vi "Example Client.vi"() -> ()   [LabVIEW 2018, in "TCPServer.lvlib"]
uses:
  TCPServer.lvlib
  TypeDefs/CCSDS.ctl
  TypeDefs/Sec Hdr CMD.ctl
  TypeDefs/Sec Hdr TLM.ctl
  d66480fc-37c9-4712-92ef-9cdd99e438f4.vi
panel:
  in  "CMD in":cluster{"U8":u8, "DBL":dbl}={"U8"=2, "DBL"=3.14}
  out "TLM out":cluster{"VOLTAGE":dbl, "NAME[20]":string}
  out "TLM Length":i32
  out "TLM Packet":string
  in  "CMD ID":u8=1
  in  "error in (no error)":errorcluster
  out "error out":errorcluster
  out "CMD Packet":string
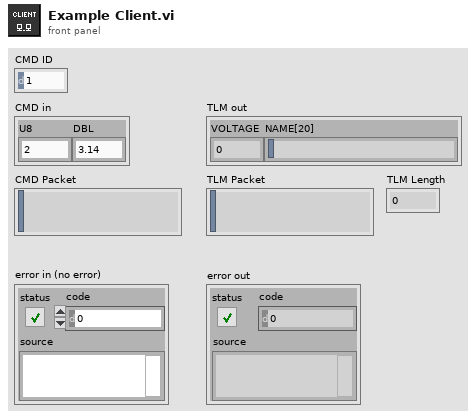
[diagram p1: front panel]
types:
  T1 = typedef "TCPServer.lvlib/Sec Hdr TLM.ctl" = cluster{"DAYS_SINCE_2000":u16, "SECONDS_SINCE_START":u32, "MS_SINCE_START":u16}
  T2 = typedef "TCPServer.lvlib/Sec Hdr CMD.ctl" = cluster{"CMD_ID":u8, "CMD_CHECKSUM":u8}
  T3 = typedef "TCPServer.lvlib/CCSDS.ctl" = cluster{"Version":u8, "Type":enum8{"TLM", "CMD"}, "SecHdrFlag":bool, "AppID":u16, "SeqFlags":u8, "SeqCount":u16, "PktLength":u16}
  T4 = cluster{"HDR_TYPE":u16, "HDR_SEQ":u16, "HDR_LENGTH":u16}
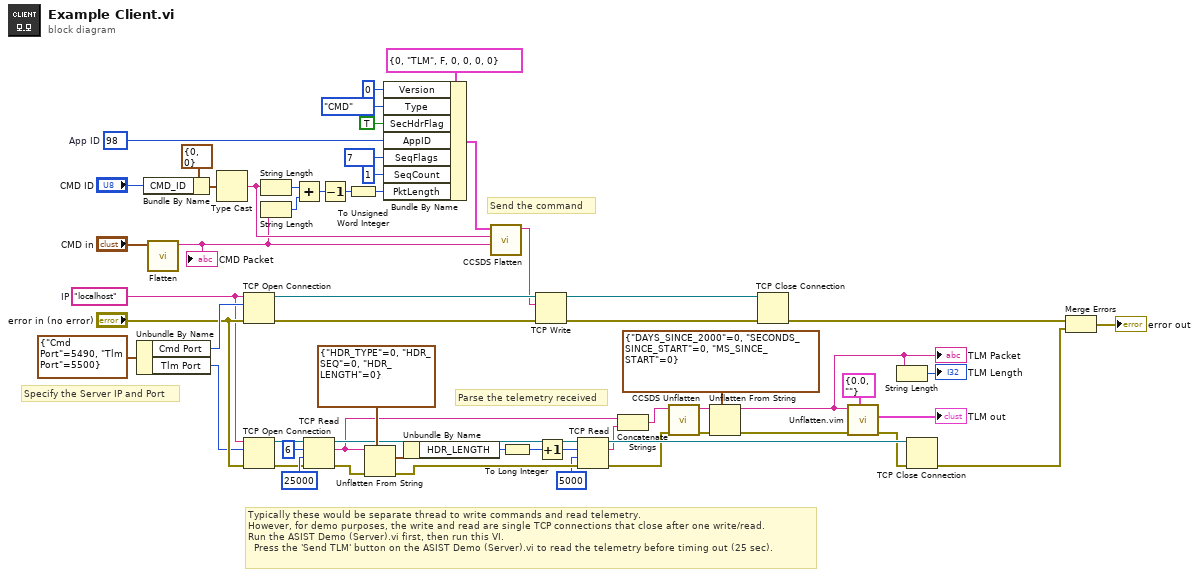
[diagram p0: block diagram]
diagram:
  w20 = u16 98  # App ID
  w16 = "localhost"  # IP
  # "Send the command"
  # "Parse the telemetry received"
  # "Typically these would be separate thread to write commands and read telemetry.\nHowever, for demo purposes, the write and read are single TCP connections that close after one write/read.\nRun the ASIST Demo (Server).vi first, then run this VI.\n  Press the 'Send TLM' button on the ASIST Demo (Server).vi to read the telemetry before timing out (25 sec)."
  # "Specify the Server IP and Port"
  n1 = Unbundle By Name(cluster{"Cmd Port":u16, "Tlm Port":u16} {"Cmd Port"=5490, "Tlm Port"=5500} ("Ports")) -> ("Cmd Port"=w18:u16, "Tlm Port"=w15:u16)
  n2 = Bundle By Name(cluster=T2 {"CMD_ID"=0, "CMD_CHECKSUM"=0} ("CCSDS Secondary Header in"), "CMD_ID"="CMD ID") -> (w32:T2)
  n3 = call "Flatten.vi"("Cluster"="CMD in") -> ("String"=w6:string)  [unwired: 9 in, 1 out]
  "CMD Packet" <- w6
  n4 = Type Cast(x=w32) -> (*(type *) &x=w31:string)  [unwired: 1 in]
  n5 = TCP Open Connection(address=w16, remote port or service name=w18, error in (no error)="error in (no error)") -> (connection ID=w59:refnum<k5>, error out=w58:errorcluster)  [unwired: 2 in]
  n6 = TCP Open Connection(address=w16, remote port or service name=w15, error in (no error)="error in (no error)") -> (connection ID=w13:refnum<k5>, error out=w14:errorcluster)  [unwired: 2 in]
  n7 = String Length(string=w31) -> (length=w37:i32)
  n8 = String Length(string=w6) -> (length=w36:i32)
  n9 = Add(x=w37, y=w36) -> (x+y=w35:i32)
  n10 = TCP Read(connection ID=w13, bytes to read=6, error in (no error)=w14, 9:25000 ("timeout ms (25000)")) -> (connection ID out=w45:refnum<k5>, data out=w43:string, error out=w53:errorcluster)  [unwired: 1 in]
  n11 = Decrement(x=w35) -> (x-1=w33:i32)
  n12 = To Unsigned Word Integer(number=w33) -> (unsigned 16bit integer=w34:u16)
  n13 = Unflatten From String(type=T4 {"HDR_TYPE"=0, "HDR_SEQ"=0, "HDR_LENGTH"=0} ("ASIST"), binary string=w43, error in (no error)=w53) -> (value=w50:T4, error out=w51:errorcluster)  [unwired: 2 in, 1 out]
  n14 = Bundle By Name(cluster=T3 {"Version"=0, "Type"=enum."TLM", "SecHdrFlag"=FALSE, "AppID"=0, "SeqFlags"=0, "SeqCount"=0, "PktLength"=0} ("CCSDS Primary Header in"), "Version"=u8 0, "Type"=enum8{"TLM", "CMD"}."CMD", "SecHdrFlag"=TRUE, "AppID"=w20, "SeqFlags"=u8 7, "SeqCount"=u16 1, "PktLength"=w34) -> (w38:T3)
  n15 = Unbundle By Name(w50) -> ("HDR_LENGTH"=w49:u16)
  n16 = call "CCSDS Flatten.vi"("Packet Data in"=w6, "Secondary Header in"=w31, "CCSDS Primary Header in"=w38) -> ("CCSDS Packet out"=w39:string)  [unwired: 7 in, 1 out]
  n17 = To Long Integer(number=w49) -> (32bit integer=w48:i32)
  n18 = TCP Write(connection ID=w59, data in=w39, error in (no error)=w58) -> (connection ID out=w11:refnum<k5>, error out=w12:errorcluster)  [unwired: 1 in, 1 out]
  n19 = Increment(x=w48) -> (x+1=w40:i32)
  n20 = TCP Read(connection ID=w45, bytes to read=w40, error in (no error)=w51, 9:5000 ("timeout ms (25000)")) -> (connection ID out=w55:refnum<k5>, data out=w44:string, error out=w42:errorcluster)  [unwired: 1 in]
  n21 = Concatenate Strings(w43, w44) -> (w41:string)
  n22 = call "CCSDS Unflatten.vi"("error in (no error)"=w42, "CCSDS Packet in"=w41) -> ("error out"=w24:errorcluster, "Remaining Data out"=w22:string)  [unwired: 7 in, 1 out]
  n23 = Unflatten From String(type=T1 {"DAYS_SINCE_2000"=0, "SECONDS_SINCE_START"=0, "MS_SINCE_START"=0} ("SecHdrTLM"), binary string=w22, error in (no error)=w24) -> (rest of the binary string=w3:string, error out=w23:errorcluster)  [unwired: 2 in, 1 out]
  "TLM Packet" <- w3
  n24 = TCP Close Connection(connection ID=w11, error in (no error)=w12) -> (error out=w10:errorcluster)  [unwired: 1 in, 1 out]
  n25 = call "Unflatten.vim"("Cluster"=cluster{"VOLTAGE":dbl, "NAME[20]":string} {"VOLTAGE"=0.0, "NAME[20]"=""} ("TLM out"), "error in (no error)"=w23, "String"=w3) -> ("error out"=w4:errorcluster, "Cluster out"=→"TLM out":cluster{"VOLTAGE":dbl, "NAME[20]":string})  [unwired: 6 in, 1 out]
  n26 = String Length(string=w3) -> (length=→"TLM Length":i32)
  n27 = TCP Close Connection(connection ID=w55, error in (no error)=w4) -> (error out=w9:errorcluster)  [unwired: 1 in, 1 out]
  n28 = Merge Errors(w10, w9) -> (→"error out":errorcluster)
